vi "Analysis.Data Dump, Meas Item Var List to 1D Str.vi"(7 "Names":string[](array[string]), 11 "MeasItems":variant) -> (3 "Data List out":string[](array[string]))   [LabVIEW 2024]
uses:
  Analysis.MeasVal.ctl
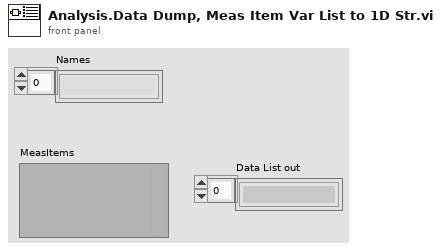
[diagram p1: front panel]
types:
  T1 = typedef "Analysis.MeasVal.ctl" = cluster{"ValStr":string, "ValNum":dbl, "Pass":bool, "Time":timestamp, "IsNum":bool}
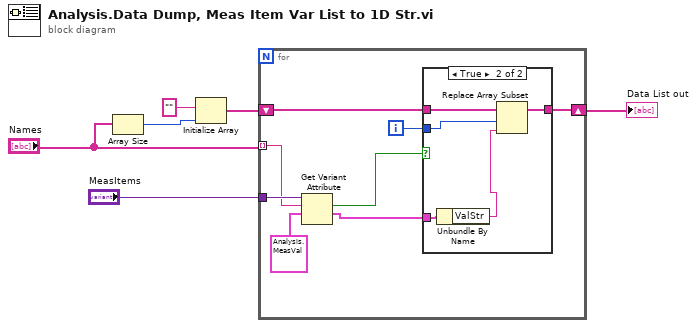
[diagram p0: block diagram]
diagram:
  n1 = Array Size(array="Names") -> (size(s)=w2:i32)
  n2 = Initialize Array("", w2) -> (w5:string[])
  n3 = for {
    tunnel: "Names" -> [w10] mode=indexing
    shift-right: [w12] -> w4
    shift-left: w5 -> [w14]
    tunnel: "MeasItems" -> [w11]
    i -> [w9]
    n4 = Get Variant Attribute(Variant=w11, name=w10, default value (empty Variant)=T1 {"ValStr"="", "ValNum"=0.0, "Pass"=FALSE, "Time"=timestamp(0 s since 1904-01-01), "IsNum"=FALSE} ("MeasValue")) -> (found=w13:bool, value=w7:T1)  [unwired: 1 in, 2 out]
    n5 = case shown="True" w13 {
      tunnel: w14 -> [w15 w20]
      tunnel: [w15 w19] -> w12
      tunnel: w9 -> [_ w18]
      tunnel: w7 -> [_ w17]
      frame False {
      }
      frame True {
        n6 = Unbundle By Name(w17) -> ("ValStr"=w16:string)
        n7 = Replace Array Subset(array=w20, new element=w16, index=w18) -> (w19:string[])
      }
    }
  }
  "Data List out" <- w4
